vi "JSON to LTRE.vi"(8 "error in (no error)":errorcluster, 11 "JSON Data In":string) -> (0 "error out":errorcluster, 2 "values":string[](array[string]), 3 "names":string[](array[string]))   [LabVIEW 2019, in "Userlib.lvlib"]
uses:
  Userlib.lvlib
  <vilib>/JDP Science/JSONtext/String Subset.vi
  <vilib>/JDP Science/JSONtext/support/Strip Quotes and Unescape.vi
  <vilib>/JDP Science/JSONtext/Parsing/Parse Full Path or Item Name.vi
  <vilib>/JDP Science/JSONtext/Offset/Find Item Locations by Path.vi
  <vilib>/JDP Science/JSONtext/support/Unescape JSON string.vi
  <vilib>/JDP Science/JSONtext/JSONtext.lvlib
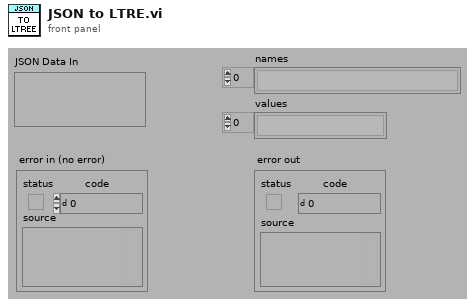
[diagram p1: front panel]
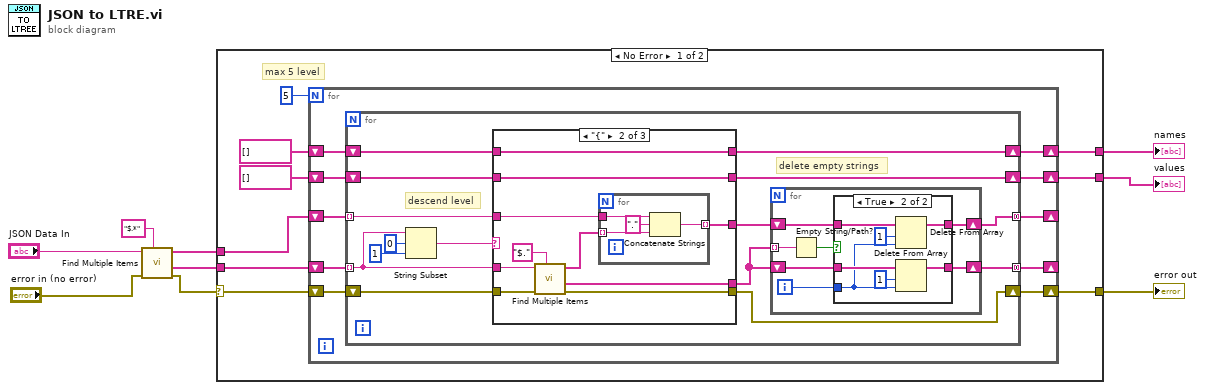
[diagram p0: block diagram]
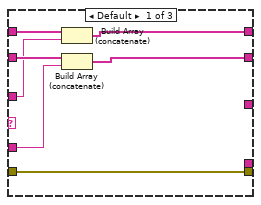
[diagram p2: hidden frame]
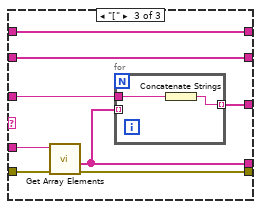
[diagram p3: hidden frame]
diagram:
  n1 = call <vilib>:"Find Multiple Items.vi"("$Path or Item Name"="$.*", "error in (no error)"="error in (no error)", "JSON"="JSON Data In") -> ("error out"=w4:errorcluster, "<JSON>"=w7:string[], "Item Names"=w6:string[])  [unwired: 5 in, 1 out]
  n2 = case shown="No Error" w4 {
    selector: w4 -> [w15 w91]
    tunnel: w7 -> [w17 _]
    tunnel: w6 -> [w14 _]
    tunnel: [w12 w91] -> w1
    tunnel: [w11 _] -> w3
    tunnel: [w10 _] -> w2
    frame No Error {
      # "max 5 level"
      n3 = for {
        N: 5 -> [_]
        shift-right: [w27] -> w10
        shift-left: string[] [] -> [w28]
        shift-right: [w24] -> _
        shift-left: w14 -> [w26]
        shift-right: [w23] -> _
        shift-left: w17 -> [w25]
        shift-right: [w21] -> w12
        shift-left: w15 -> [w22]
        shift-right: [w20] -> w11
        shift-left: string[] [] -> [w19]
        n4 = for {
          shift-right: [w40] -> w27
          shift-left: w28 -> [w43]
          tunnel: [w36] -> w24 mode=concatenating
          tunnel: [w35] -> w23 mode=concatenating
          tunnel: w26 -> [w39] mode=indexing
          tunnel: w25 -> [w38] mode=indexing
          shift-right: [w32] -> w21
          shift-left: w22 -> [w33]
          shift-right: [w31] -> w20
          shift-left: w19 -> [w30]
          # "delete empty strings"
          # "descend level"
          n5 = String Subset(string=w38, offset (0)=0, length (rest)=1 ("length (rest)")) -> (substring=w29:string)
          n6 = case shown="\"{\"" w29 {
            tunnel: w38 -> [w48 w58 w68]
            tunnel: w39 -> [w44 w57 w71]
            tunnel: w43 -> [w50 w60 w72]
            tunnel: [w49 w60 w72] -> w40
            tunnel: [_ w56 w65] -> w37
            tunnel: [_ w52 w70] -> w34
            tunnel: w33 -> [w47 w54 w67]
            tunnel: [w47 w53 w66] -> w32
            tunnel: [w45 w51 w69] -> w31
            tunnel: w30 -> [w46 w51 w69]
            frame Default {
              n7 = Build Array (concatenate)(w46, w44) -> (w45:string[])
              n8 = Build Array (concatenate)(w50, w48) -> (w49:string[])
            }
            frame "{" {
              n9 = call <vilib>:"Find Multiple Items.vi"("$Path or Item Name"="$.", "error in (no error)"=w54, "JSON"=w58) -> ("error out"=w53:errorcluster, "<JSON>"=w56:string[], "Item Names"=w55:string[])  [unwired: 5 in, 1 out]
              n10 = for {
                tunnel: w55 -> [w61] mode=indexing
                tunnel: w57 -> [w64]
                tunnel: [w62] -> w52 mode=indexing
                n11 = Concatenate Strings(w64, "." ("string"), w61) -> (w62:string)
              }
            }
            frame "[" {
              n12 = call <vilib>:"Get Array Elements.vi"("error in (no error)"=w67, "JSON"=w68) -> ("error out"=w66:errorcluster, "<JSON>"=w65:string[])  [unwired: 7 in, 1 out]
              n13 = for {
                tunnel: w71 -> [w74]
                tunnel: [w73] -> w70 mode=indexing
                tunnel: w65 -> [_] mode=indexing
                n14 = Concatenate Strings(w74) -> (w73:string)
              }
            }
          }
          n15 = for {
            shift-right: [w76] -> w36
            shift-left: w34 -> [w78]
            shift-right: [w75] -> w35
            shift-left: w37 -> [w77]
            tunnel: w37 -> [w81] mode=indexing
            i -> [w79]
            n16 = Empty String/Path?(string/path=w81) -> (empty?=w80:bool)
            n17 = case shown="True" w80 {
              tunnel: w79 -> [_ w84]
              tunnel: w78 -> [w83 w90]
              tunnel: w77 -> [w82 w87]
              tunnel: [w83 w86] -> w76
              tunnel: [w82 w85] -> w75
              frame False {
              }
              frame True {
                n18 = Delete From Array(array=w90, length=1, index=w84) -> (array with subset deleted=w86:string[])  [unwired: 1 out]
                n19 = Delete From Array(array=w87, length=1, index=w84) -> (array with subset deleted=w85:string[])  [unwired: 1 out]
              }
            }
          }
        }
      }
    }
    frame Error {
    }
  }
  "error out" <- w1
  "names" <- w3
  "values" <- w2
